vi "MainRT_APA.vi"() -> ()   [LabVIEW 2019]
uses:
  <vilib>/Platform/TimedLoop/XDataNode/wakeup.ctl
  <vilib>/Platform/TimedLoop/XDataNode/XDNodeRunTimeDep.lvlib
  <vilib>/Platform/TimedLoop/XDataNode/nitl_modes.ctl
  <vilib>/Platform/TimedLoop/XDataNode/timing_clust.ctl
  <vilib>/platform/TimedLoop/XDataNode/XDataNode.xnode
  <vilib>/rvi/interface/nirviReadWriteControl/nirviReadWriteControl.xnode
  <vilib>/myRIO/Instrument Drivers/Onboard IO/UART/typedef/VISA Configuration.ctl
  <vilib>/myRIO/Instrument Drivers/Onboard IO/UART/UART.lvlib
  <vilib>/rvi/interface/nirviOpenFPGA/nirviOpenFPGA.xnode
  NiFpgaLv.dll
  <vilib>/Utility/error.llb/Error Cluster From Error Code.vi
  <vilib>/rvi/interface/Simulation/niFpgaSimulationCallBeginRW.vi
  <vilib>/rvi/errors/niLvFpgaAdjustHostInterfaceError.vi
  <vilib>/rvi/interface/nirviCloseFPGA/nirviCloseFPGA.xnode
  <vilib>/FPGAPlugInAG/Dynamic/niLvFpga_Close_Dynamic.vi
  <vilib>/Instr/_visa.llb/VISA Configure Serial Port (Instr).vi
  FPGA Bitfiles/apa_FPGATarget_MainFPGAAPA_fCWPdocsT-Y.lvbitx
  MainFPGA_APA.vi
  <vilib>/FPGAPlugInAG/myRIO-1900/niLvFpga_Open_myRIO-1900.vi
  <vilib>/rvi/interface/common/dynamic/niFpgaDynamicAddResources.vi
panel:
  out "Waveform Chart":cluster{dbl, dbl, "Gyro_z":dbl}(graph)
  in  "Period":i64=1
  out "Latency":i16
  in  "error in":errorcluster
  in  "file no.":u32
  out "error out":errorcluster
  in  "stop":bool
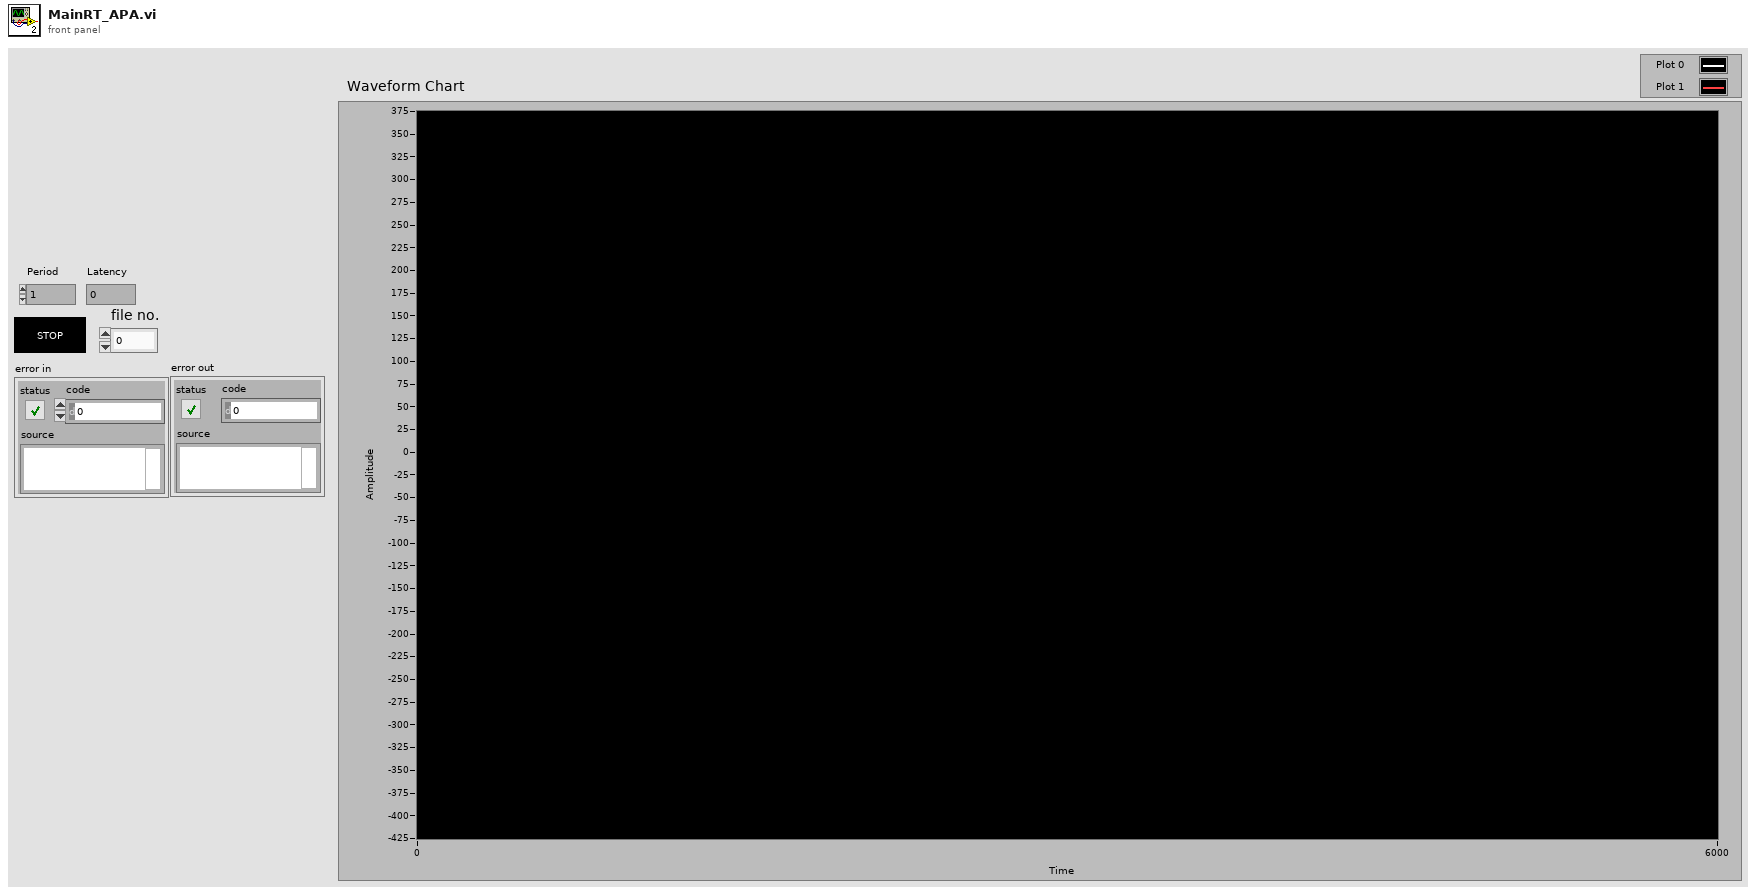
[diagram p1: front panel]
types:
  T1 = typedef "UART.lvlib/VISA Configuration.ctl" = cluster{"baud rate (9600)":u32, "data bits (8)":u16, "parity (0:none)":enum16{"None", "Odd", "Even", "Mark", "Space"}, "stop bits (10: 1 bit)":u16, "flow control (0:none)":u16, "termination char\n(0xA = '\\n' = LF) ":u8, "Enable Termination\nChar (T)":bool, "timeout (10sec)":u32}
  T2 = enum16{"open", "replace", "create", "open or create", "replace or create", "replace or create with confirmation"}
  T3 = typedef "XDNodeRunTimeDep.lvlib/timing_clust.ctl" = cluster{"Expected End [f-1]":u64, "Actual End [f-1]":u64, "Finished Late? [f-1]":bool, "Expected End [i-1]":u64, "Actual End [i-1]":u64, "Finished Late? [i-1]":bool, "Expected Start [i]":u64, "Actual Start [i]":u64, "Expected Start [f]":u64, "Actual Start [f]":u64, "Source Name":string, "Structure Name":string, "Period":i64, "Deadline":i64, "Offset":i64, "Start":i64, "Priority":i32, "Timeout":i32, "Mode":T4, "Wakeup Reason":T5, "Error":errorcluster, "Source Type":string, "Secondary Source Type":string, "Global End Time":u64, "Global Start Time":u64, "Frame Duration":u64, "Iteration Duration":u64, "Assigned CPU":i32, "I/O Scan Engine Mode":u32}
  T4 = typedef "XDNodeRunTimeDep.lvlib/nitl_modes.ctl" = enum32{"No Change", "Process missed periods, maintain original phase", "Discard missed periods, maintain original phase", "Process missed periods, ignore original phase", "Discard missed periods, ignore original phase"}
  T5 = typedef "XDNodeRunTimeDep.lvlib/wakeup.ctl" = enum32{"Normal", "Aborted", "Asynchronous wakeup", "Timing source error", "Timed loop error", "Timeout"}
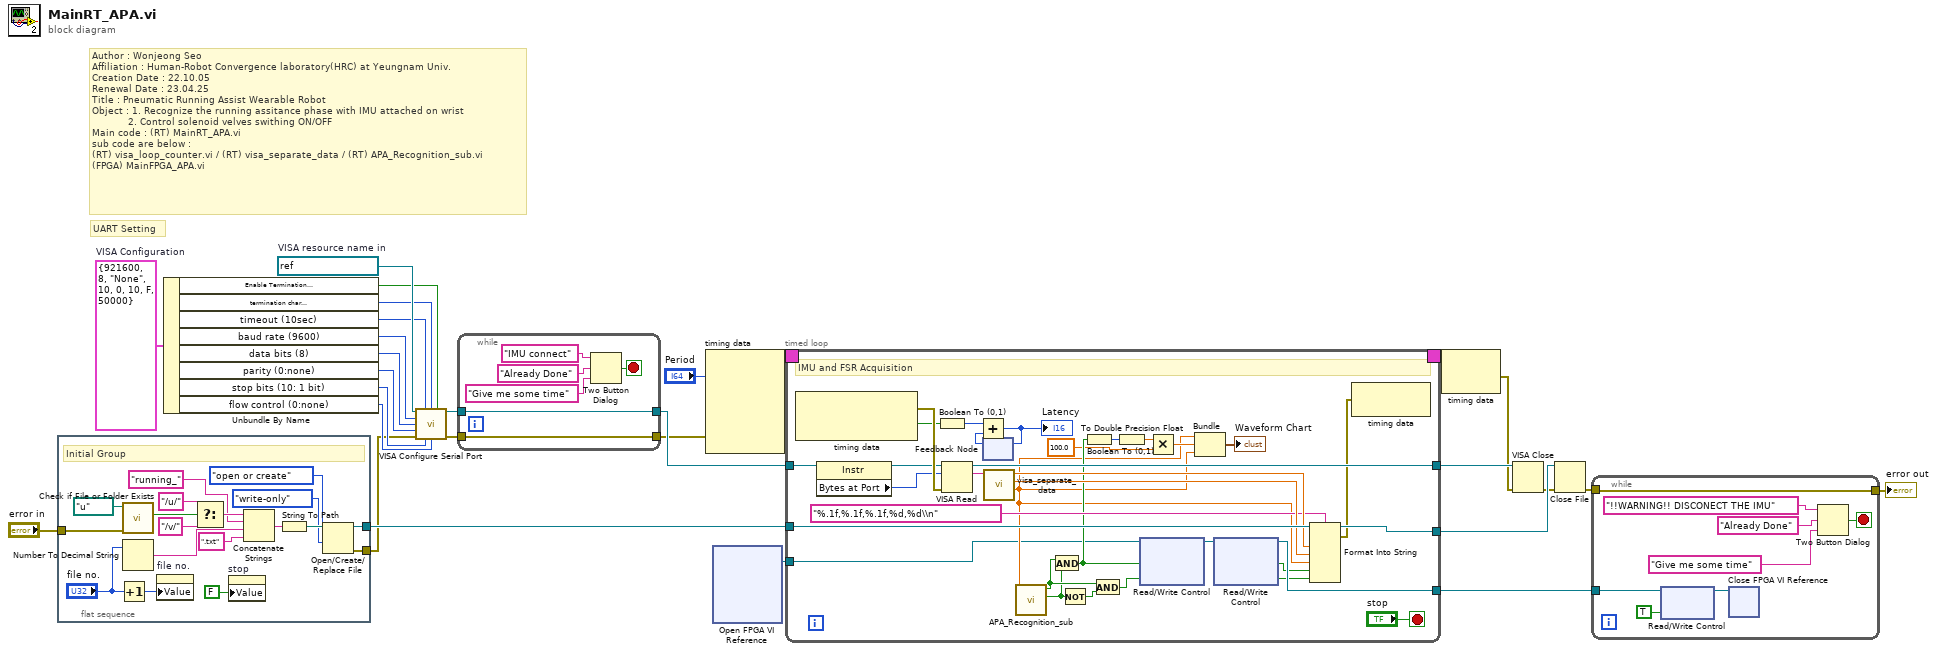
[diagram p0: block diagram]
diagram:
  w25 = T1 {"baud rate (9600)"=921600, "data bits (8)"=8, "parity (0:none)"=enum."None", "stop bits (10: 1 bit)"=10, "flow control (0:none)"=0, "termination char\n(0xA = '\\n' = LF) "=10, "Enable Termination\nChar (T)"=FALSE, "timeout (10sec)"=50000}  # VISA Configuration
  w26 = refnum<visa-resource-name> "ASRL1::INSTR"  # VISA resource name in
  # "Author : Wonjeong Seo\nAffiliation : Human-Robot Convergence laboratory(HRC) at Yeungnam Univ.\nCreation Date : 22.10.05\nRenewal Date : 23.04.25\nTitle : Pneumatic Running Assist Wearable Robot\nObject : 1. Recognize the running assitance phase with IMU attached on wrist\n            2. Control solenoid velves swithing ON/OFF\nMain code : (RT) MainRT_APA.vi\nsub code are below :\n(RT) visa_loop_counter.vi / (RT) visa_separate_data / (RT) APA_Recognition_sub.vi\n(FPGA) MainFPGA_APA.vi"
  # "UART Setting"
  n1 = flat-sequence {
    tunnel: "error in" -> [w30]
    tunnel: [w31] -> w5
    tunnel: [w29] -> w4
    frame #0 {
      # "Initial Group"
      n2 = Increment(x="file no.") -> (x+1=w44:u32)
      n3 = call <vilib>:"Check if File or Folder Exists.vi"("error in (no error)"=w30, "path"=path "u:/") -> ("file or folder exists?"=w39:bool)  [unwired: 7 in, 2 out]
      n4 = Number To Decimal String(number="file no.") -> (decimal integer string=w43:string)  [unwired: 1 in]
      n5 = property on="file no." class="DigNum (strict)"("Value"=w44) -> ()  [unwired: 2 in, 2 out]
      n6 = Select(t="/u/", s=w39, f="/v/") -> (s? t:f=w41:string)
      n7 = property on="stop" class="Bool (strict)"("Value"=FALSE ("stop")) -> ()  [unwired: 2 in, 2 out]
      n8 = Concatenate Strings(w41, "running_" ("string"), w43, ".txt" ("string")) -> (w42:string)
      n9 = String To Path(string=w42) -> (path=w40:path)
      n10 = Open/Create/Replace File(file path (use dialog)=w40, operation (0:open)=T2."open or create", access (0:read/write)=enum16{"read/write", "read-only", "write-only"}."write-only") -> (refnum out=w31:refnum<file>, error out=w29:errorcluster)  [unwired: 3 in, 1 out]
    }
  }
  n11 = Unbundle By Name(w25) -> ("Enable Termination\nChar (T)"=w24:bool, "termination char\n(0xA = '\\n' = LF)"=w23:u8, "timeout (10sec)"=w22:u32, "baud rate (9600)"=w18:u32, "data bits (8)"=w19:u16, "parity (0:none)"=w20:enum16{"None", "Odd", "Even", "Mark", "Space"}, "stop bits (10: 1 bit)"=w21:u16, "flow control (0:none)"=w17:u16)
  n12 = call-poly "VISA Configure Serial Port"("VISA resource name"=w26, "timeout (10sec)"=w22, "termination char\n(0xA = '\\n' = LF)"=w23, "Enable Termination\nChar (T)"=w24, "baud rate (9600)"=w18, "data bits (8)"=w19, "parity (0:none)"=w20, "error in (no error)"=w4, "stop bits (10: 1 bit)"=w21, "flow control (0:none)"=w17) -> ("VISA resource name out"=w14:refnum<visa-resource-name>, "error out"=w13:errorcluster)  [unwired: 4 in]
  n13 = while {
    tunnel: [w52] -> w10
    tunnel: w13 -> [w52]
    tunnel: [w51] -> w12
    tunnel: w14 -> [w51]
    stop <- w47 stop-if-true
    n14 = Two Button Dialog(message="IMU connect", 1:"Give me some time" ("F button name (\"Cancel\")"), 2:"Already Done" ("button name (\"OK\")")) -> (T button?=w47:bool)
  }
  n15 = node-c288("Period", w10) -> (w28:T3)  [unwired: 3 in]
  n16 = xnode ("Open FPGA VI Reference")() -> ("FPGA VI Reference Out"=w9:refnum<k20>)  [unwired: 2 in, 1 out]
  n17 = timed-loop {
    timing: w28 -> [_]
    timing-out: [_] -> w27
    tunnel: w12 -> [w81]
    tunnel: [w85] -> w16
    tunnel: w9 -> [w53]
    tunnel: [w75] -> w3
    tunnel: w5 -> [w78]
    tunnel: [w77] -> w8
    stop <- "stop" stop-if-true
    # "IMU and FSR Acquisition"
    n18 = node-c288() -> (w83:errorcluster, w69:bool)  [unwired: 1 in]
    n19 = property class="Instr"(reference=w81) -> (reference out=w80:refnum<visa-resource-name>, "Bytes at Port"=w79:u32)  [unwired: 1 in, 1 out]
    n20 = Boolean To (0,1)(Boolean=w69) -> (0, 1=w68:i16)
    n21 = VISA Read(VISA resource name=w80, byte count=w79, error in (no error)=w83) -> (VISA resource name out=w85:refnum<visa-resource-name>, read buffer=w84:string)  [unwired: 2 out]
    n22 = feedback #1() -> (w66:i16)  [unwired: 1 in]
    n23 = Add(x=w68, y=w66) -> (x+y=w67:i16)
    "Latency" <- w67
    n24 = feedback-in #1(w67) -> ()
    n25 = call "visa_separate_data.vi"("Input string"=w84) -> ("Gyro_z"=w60:dbl, "Gyro_y"=w72:dbl, "Gyro_x"=w73:dbl)  [unwired: 7 in, 1 out]
    n26 = call "APA_Recognition_sub.vi"("IMU_IN[k]"=w60) -> ("Same Sagittal Direction"=w56:bool, "Assist Reference"=w58:bool)  [unwired: 8 in, 1 out]
    n27 = And(x=w58, y=w56) -> (x .and. y?=w64:bool)
    n28 = Not(x=w56) -> (.not. x?=w57:bool)
    n29 = Boolean To (0,1)(Boolean=w64) -> (0, 1=w54:i16)
    n30 = And(x=w58, y=w57) -> (x .and. y?=w59:bool)
    n31 = To Double Precision Float(number=w54) -> (double precision float=w55:dbl)
    n32 = xnode "Read/Write Control"("FPGA VI Reference In"=w53, "A_Digit0"=w64, "A_Digit3"=w59) -> ("FPGA VI Reference Out"=w74:refnum<k20>)  [unwired: 1 in, 1 out]
    n33 = Multiply(x=w55, y=100.0) -> (x*y=w62:dbl)
    n34 = Bundle("Gyro_z"=w60, w62, "Gyro_z"=w60) -> (→"Waveform Chart":cluster{"Gyro_z":dbl, dbl, "Gyro_z":dbl})  [unwired: 1 in]
    n35 = xnode "Read/Write Control"("FPGA VI Reference In"=w74) -> ("FPGA VI Reference Out"=w75:refnum<k20>, "A_Digit0"=w65:bool, "A_Digit3"=w71:bool)  [unwired: 1 in, 1 out]
    n36 = Format Into String(format string="%.1f,%.1f,%.1f,%d,%d\\n", initial string=w78, w73, w72, w60, w65, w71) -> (resulting string=w77:refnum<file>, error out=w76:errorcluster)  [unwired: 1 in]
    n37 = node-c288(w76) -> ()  [unwired: 1 out]
  }
  n38 = node-c288(w27) -> (w7:errorcluster)
  n39 = VISA Close(VISA resource name=w16, error in (no error)=w7) -> (error out=w6:errorcluster)
  n40 = Close File(refnum=w8, error in=w6) -> (error out=w2:errorcluster)  [unwired: 1 out]
  n41 = while {
    tunnel: [w99] -> w15
    tunnel: w2 -> [w99]
    tunnel: w3 -> [w94]
    stop <- w95 stop-if-true
    n42 = xnode "Read/Write Control"("FPGA VI Reference In"=w94, "stop"=TRUE) -> ("FPGA VI Reference Out"=w92:refnum<k20>)  [unwired: 1 in, 1 out]
    n43 = xnode "Close FPGA VI Reference"("FPGA VI Reference In"=w92) -> ()  [unwired: 1 in, 1 out]
    n44 = Two Button Dialog(message="!!WARNING!! DISCONECT THE IMU", 1:"Give me some time" ("F button name (\"Cancel\")"), 2:"Already Done" ("button name (\"OK\")")) -> (T button?=w95:bool)
  }
  "error out" <- w15
